vi "Parse Light IDs.vi"(8 "error in":errorcluster, 10 "Light JSON":string="{\"1\":{\"name\": \"Hue Lamp\"},\"2\":{\"name\": \"Hue Lamp 1\"},\"3\":{\"name\": \"Hue Lamp 2\"}}") -> (0 "error out":errorcluster, 1 "Light Data":string[](array[string]), 2 "Light IDs":i32[](array[numeric]))   [LabVIEW 2020, in "LMH-Hue.lvlib"]
uses:
  LMH-Hue.lvlib
  <vilib>/JDP Science/JSONtext/JSONtext.lvlib
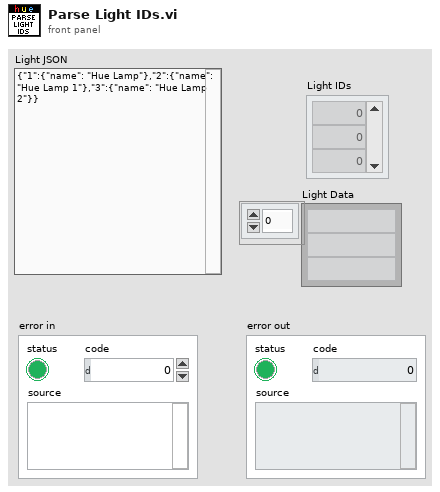
[diagram p1: front panel]
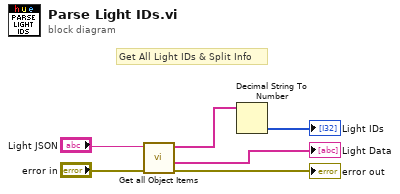
[diagram p0: block diagram]
diagram:
  # "Get All Light IDs & Split Info"
  n1 = call <vilib>:"Get all Object Items.vi"("error in (no error)"="error in", "JSON"="Light JSON") -> ("error out"=→"error out":errorcluster, "<JSON>"=→"Light Data":string[], "Item Names"=w6:string[])  [unwired: 6 in, 1 out]
  n2 = Decimal String To Number(string=w6) -> (number=→"Light IDs":i32[])  [unwired: 2 in, 1 out]
